vi "Main.vi"(11 "Module Admin":refnum<class "Delacor_lib_QMH_Cloneable Module Admin.lvclass">) -> ()   [LabVIEW 2020, in "Monochromator.lvlib"]
doc: "This template is based off of the Queued Message Handler design pattern and the Queued Message Handler project template that ships with LabVIEW.\n\nThe main difference is that the queue is private to this module and communication between modules is performed via Broadcast and Request events.\n\nRequest events are wrapped in public API methods and are handled in the Event Handling Loop (EHL) of this VI. Any module can register for Broadcast events sent by this module. The EHL generates messages based on user interface actions.\n\nThe Message Handling Loop (MHL) processes messages generated by the EHL, or by other messages. The messages are string values, so new messages can be added easily to the Message Cases case structure in the MHL. Each message cluster can also provide an optional value for Message Data, which is a variant that can be converted to whatever message-specific data is required.\n_____\nBased on DQMH Project Template 6.1.0.94.\n____\nPantherLAB Templates 1.0.0.1\nCopyright (c) 2022, PantherLAB\n____\nPantherLAB Templates 1.0.0.5\nCopyright (c) 2022, PantherLAB"
uses:
  Monochromator.lvlib
  <vilib>/Delacor/Delacor QMH/Libraries/Cloneable Module Admin_class/Delacor_lib_QMH_Cloneable Module Admin.lvclass
  C:/Program Files (x86)/National Instruments/LabVIEW 2020/vi.lib/Delacor/Delacor QMH/Libraries/Module Admin_class/Delacor_lib_QMH_Module Admin.lvclass
  Module Data--cluster.ctl
  <vilib>/Delacor/Delacor QMH/Libraries/Cloneable Module Admin_class/Delacor_lib_QMH_Cloneable Module Admin.lvclass/Delacor_lib_QMH_Cloneable Module Admin.ctl
  Helper Loop Status--enum.ctl
  <vilib>/Delacor/Delacor QMH/Libraries/Message Queue_class/Delacor_lib_QMH_Message Queue.lvclass/Delacor_lib_QMH_Message Queue.ctl
  Stop Argument--cluster.ctl
  <vilib>/Delacor/Delacor QMH/Libraries/Module Admin_class/Delacor_lib_QMH_Module Admin.lvclass/Delacor_lib_QMH_Module Admin.ctl
  Draw Panel into Subpanel Argument--cluster.ctl
  Remove Panel from Subpanel Argument--cluster.ctl
  Connect Argument--cluster.ctl
  Connect (Reply Payload)--cluster.ctl
  Move Argument--cluster.ctl
  Read continuously Argument--cluster.ctl
  Stop continous reading Argument--cluster.ctl
  Stop movement Argument--cluster.ctl
  Ask position Argument--cluster.ctl
  Ask position (Reply Payload)--cluster.ctl
  Position reached Argument--cluster.ctl
  Position reached (Reply Payload)--cluster.ctl
  Set speed Argument--cluster.ctl
  Get speed Argument--cluster.ctl
  Get speed (Reply Payload)--cluster.ctl
  Disconnect Argument--cluster.ctl
  Move (GOTO) Argument--cluster.ctl
  Move (GOTO) (Reply Payload)--cluster.ctl
  <vilib>/Utility/miscctls.llb/LVPointTypeDef.ctl
  Support/HL Data.ctl
  <vilib>/Instr/_visa.llb/VISA Flush IO Buffer Mask.ctl
  <vilib>/Delacor/Delacor QMH/Libraries/Cloneable Module Admin_class/Delacor_lib_QMH_Get Module ID.vi
  <vilib>/Delacor/Delacor QMH/Libraries/Message Queue_class/Delacor_lib_QMH_Enqueue Message (Single).vi
  <vilib>/Delacor/Delacor QMH/Libraries/Module Admin_class/Delacor_lib_QMH_Get External Launch.vi
  <vilib>/Utility/error.llb/Error Cluster From Error Code.vi
  <vilib>/ErrorRing/Error Ring.xnode
  <vilib>/Delacor/Delacor QMH/Libraries/Message Queue_class/Delacor_lib_QMH_Message Queue.lvclass
  Local Events/Local Events.lvlib
panel:
  out "error out":errorcluster
  out "Status":string
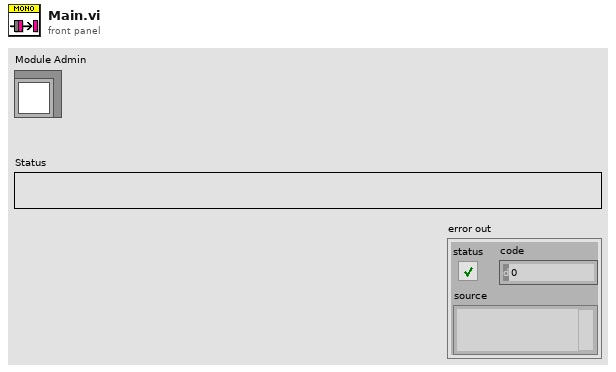
[diagram p1: front panel]
types:
  T1 = typedef "Monochromator.lvlib/Request Events--cluster.ctl" = cluster{"Stop Module":refnum<user-event>, "Show Panel":refnum<user-event>, "Hide Panel":refnum<user-event>, "Show Diagram":refnum<user-event>, "Get Module Execution Status":refnum<user-event>, "Draw Panel into Subpanel":refnum<user-event>, "Remove Panel from Subpanel":refnum<user-event>, "Connect":refnum<user-event>, "Move":refnum<user-event>, "Read continuously":refnum<user-event>, "Stop continous reading":refnum<user-event>, "Stop movement":refnum<user-event>, "Ask position":refnum<user-event>, "Position reached":refnum<user-event>, "Set speed":refnum<user-event>, "Get speed":refnum<user-event>, "Disconnect":refnum<user-event>, "Move (GOTO)":refnum<user-event>}
  T2 = typedef "Monochromator.lvlib/Local Events.lvlib/Local Events--cluster.ctl" = cluster{"Wake up Helper Loop":refnum<user-event>, "Put Helper Loop to Sleep":refnum<user-event>}
  T3 = typedef "Monochromator.lvlib/Module Data--cluster.ctl" = cluster{"Status":string, "SubPanel":refnum<vi>, "Panel Status":bool, "VISA resource name":refnum<visa-resource-name>, "Simulate?":bool, "Current position":dbl, "Current speed":dbl, "Connected?":bool, "Desired position":dbl}
  T4 = enum32{"invalid lock state", "Not Locked", "Locked (No Password)", "Password-protected"}
  T5 = typedef "Monochromator.lvlib/Stop Argument--cluster.ctl" = cluster{"Module ID":i32, "Origin":string, "Exit via Stop Module Req?":bool, "Wait for Module to stop?":bool}
  T6 = typedef "Monochromator.lvlib/Draw Panel into Subpanel Argument--cluster.ctl" = cluster{"Module ID":i32, "Sub Panel":refnum<vi>}
  T7 = typedef "Monochromator.lvlib/Remove Panel from Subpanel Argument--cluster.ctl" = cluster{"Module ID":i32, "Boolean":bool}
  T8 = typedef "Monochromator.lvlib/Connect Argument--cluster.ctl" = cluster{"Module ID":i32, "VISA resource name":refnum<visa-resource-name>, "Port config":cluster{"baud rate":u32, "data bits":u16, "parity":enum16{"None", "Odd", "Even", "Mark", "Space"}, "stop bits":u16}, "Wait Notifier":refnum<notifier>, "wait for reply":bool, "Simulate?":bool}
  T9 = typedef "Monochromator.lvlib/Move Argument--cluster.ctl" = cluster{"Module ID":i32, "Wavelength":dbl}
  T10 = typedef "Monochromator.lvlib/Read continuously Argument--cluster.ctl" = cluster{"Module ID":i32, "Timeout":i32}
  T11 = typedef "Monochromator.lvlib/Stop continous reading Argument--cluster.ctl" = cluster{"Module ID":i32, "Boolean":bool}
  T12 = typedef "Monochromator.lvlib/Stop movement Argument--cluster.ctl" = cluster{"Module ID":i32, "Boolean":bool}
  T13 = typedef "Monochromator.lvlib/Ask position Argument--cluster.ctl" = cluster{"Module ID":i32, "Wait Notifier":refnum<notifier>, "wait for reply":bool}
  T14 = typedef "Monochromator.lvlib/Position reached Argument--cluster.ctl" = cluster{"Module ID":i32, "Wait Notifier":refnum<notifier>, "wait for reply":bool}
  T15 = typedef "Monochromator.lvlib/Set speed Argument--cluster.ctl" = cluster{"Module ID":i32, "nm/min":dbl}
  T16 = typedef "Monochromator.lvlib/Get speed Argument--cluster.ctl" = cluster{"Module ID":i32, "Wait Notifier":refnum<notifier>, "wait for reply":bool}
  T17 = typedef "Monochromator.lvlib/Disconnect Argument--cluster.ctl" = cluster{"Module ID":i32, "Boolean":bool}
  T18 = typedef "Monochromator.lvlib/Move (GOTO) Argument--cluster.ctl" = cluster{"Module ID":i32, "Position":dbl, "Echo?":bool, "Wait Notifier":refnum<notifier>, "wait for reply":bool}
  T19 = typedef "LVPointTypeDef.ctl" = cluster{"Horizontal":i16, "Vertical":i16}
  T20 = enum32{"Invalid", "Standard", "Closed", "Hidden", "Minimized", "Maximized"}
  T21 = typedef "Monochromator.lvlib/Connect (Reply Payload)--cluster.ctl" = cluster{"Connected?":bool, "error":errorcluster}
  T22 = typedef "Monochromator.lvlib/Move (GOTO) (Reply Payload)--cluster.ctl" = cluster{"error":errorcluster}
  T23 = typedef "Monochromator.lvlib/HL Data.ctl" = cluster{"Helper Loop Timeout":i32, "VISA resource name":refnum<visa-resource-name>, "Module ID":i32}
  T24 = typedef "Monochromator.lvlib/Ask position (Reply Payload)--cluster.ctl" = cluster{"Current position":dbl, "error":errorcluster}
  T25 = typedef "Monochromator.lvlib/Position reached (Reply Payload)--cluster.ctl" = cluster{"Done?":bool, "error":errorcluster}
  T26 = typedef "Monochromator.lvlib/Get speed (Reply Payload)--cluster.ctl" = cluster{"nm/min":dbl, "error":errorcluster}
  T27 = typedef "Monochromator.lvlib/Helper Loop Status--enum.ctl" = enum16{"Awake", "Asleep"}
  T28 = cluster{"baud rate":u32, "data bits":u16, "parity":enum16{"None", "Odd", "Even", "Mark", "Space"}, "stop bits":u16}
  T29 = typedef "VISA Flush IO Buffer Mask.ctl" = u16
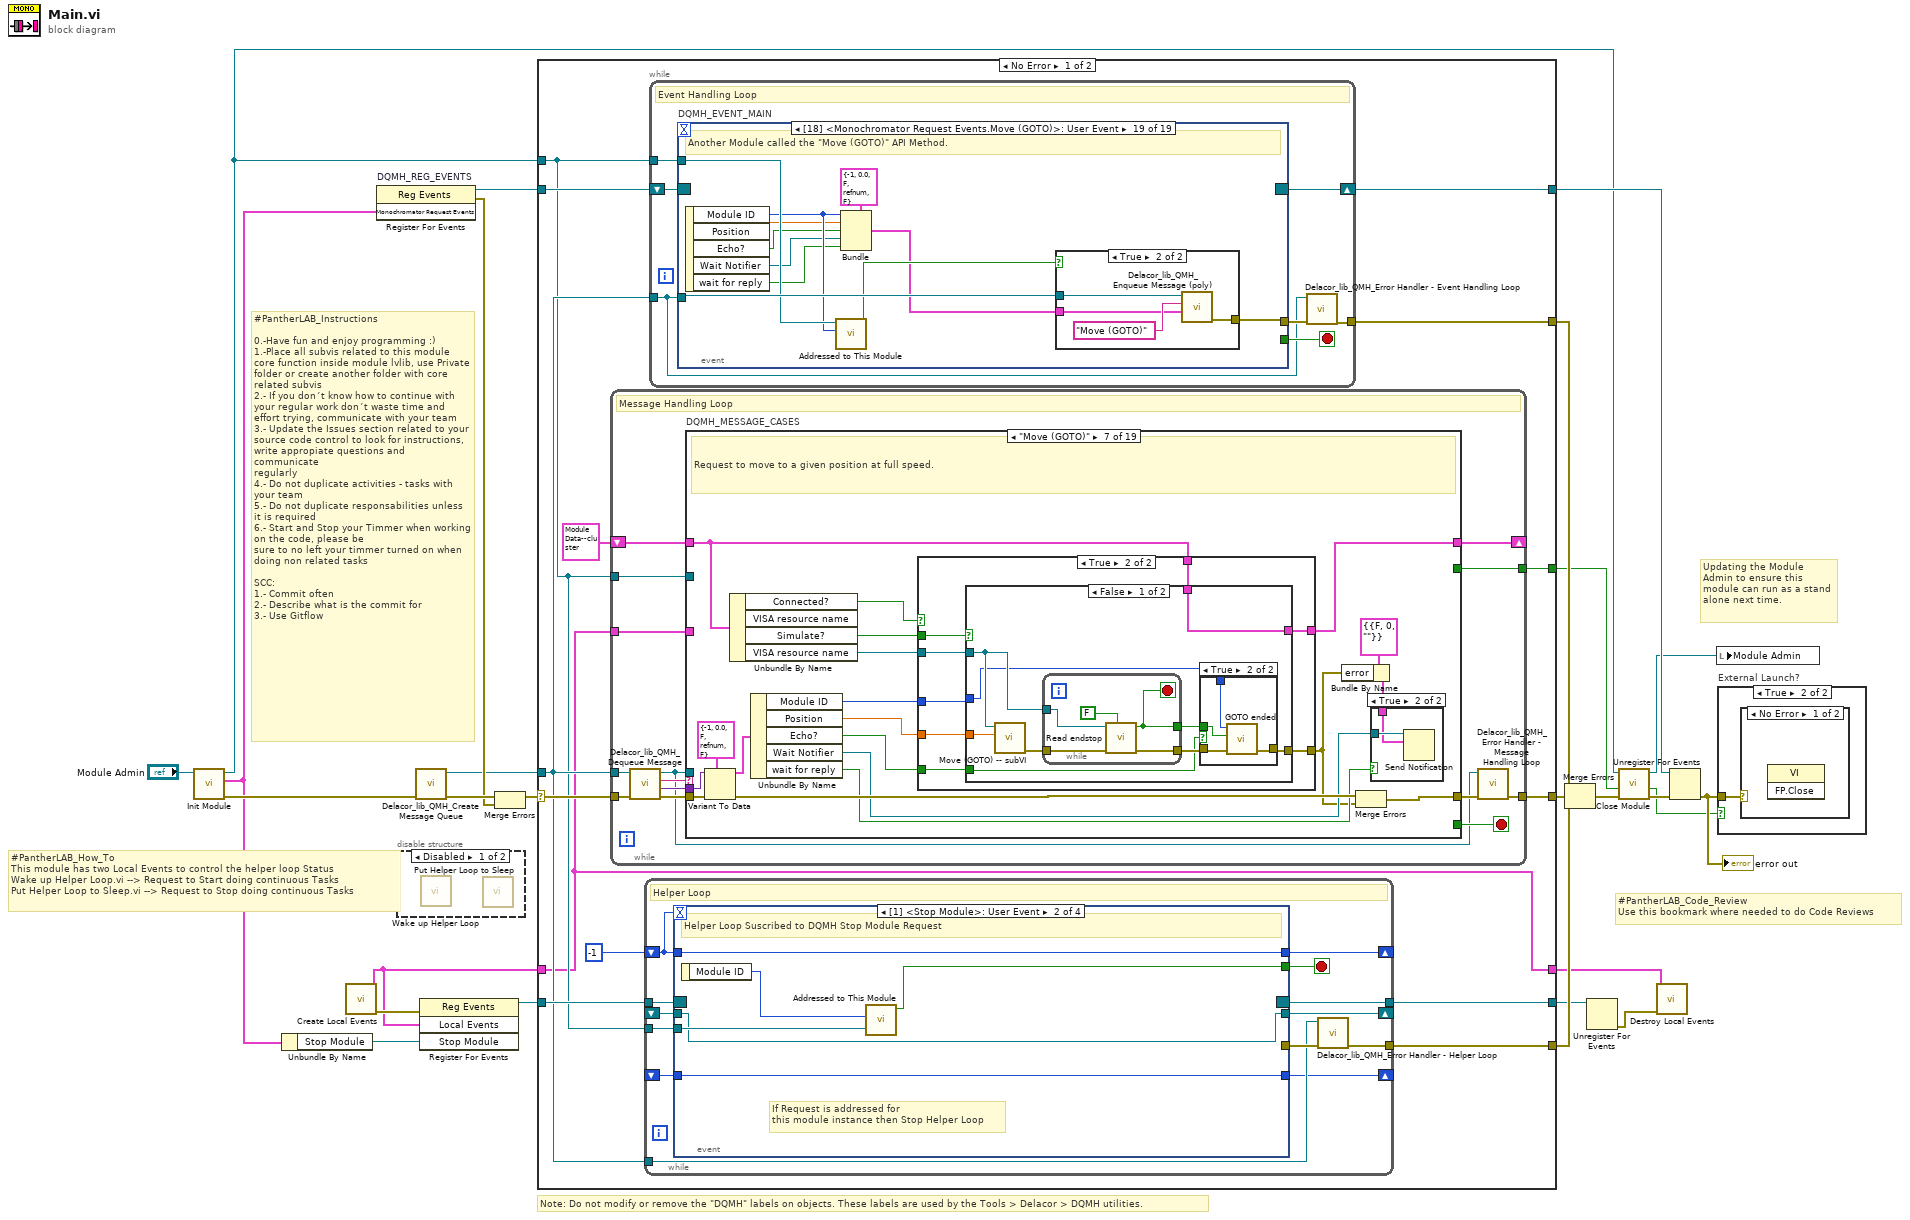
[diagram p0: block diagram]
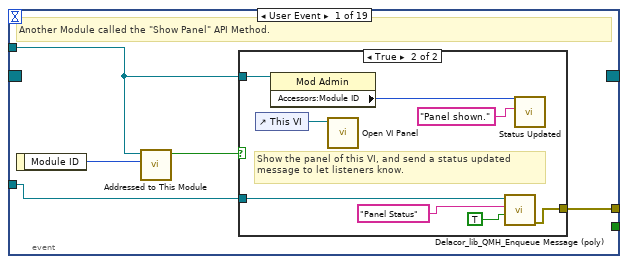
[diagram p2: hidden frame]
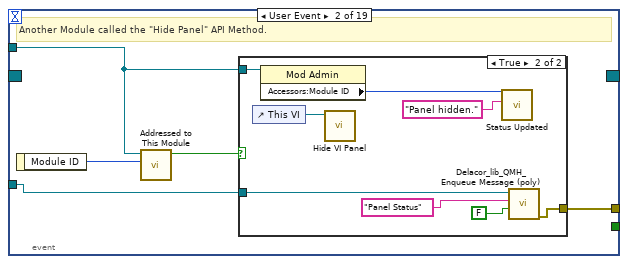
[diagram p4: hidden frame]
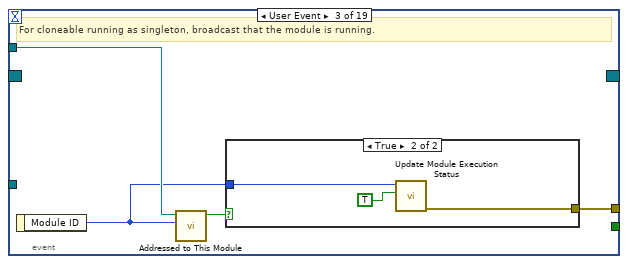
[diagram p6: hidden frame]
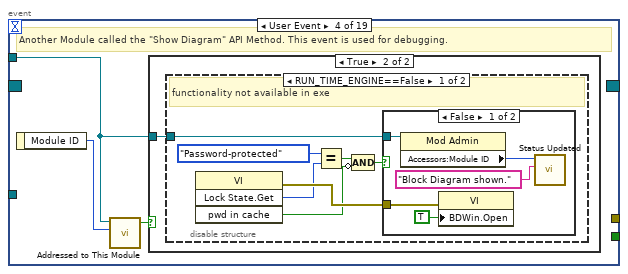
[diagram p8: hidden frame]
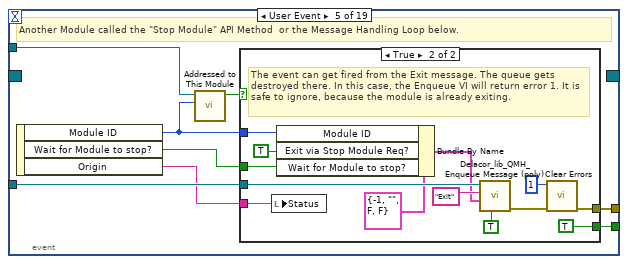
[diagram p12: hidden frame]
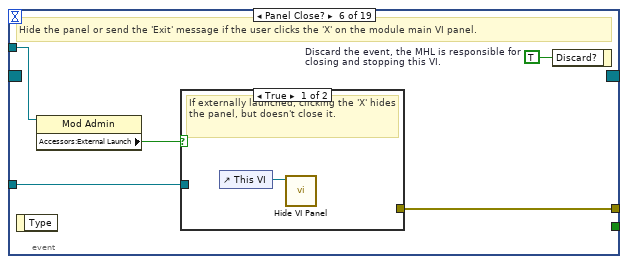
[diagram p14: hidden frame]
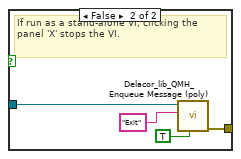
[diagram p15: hidden frame]
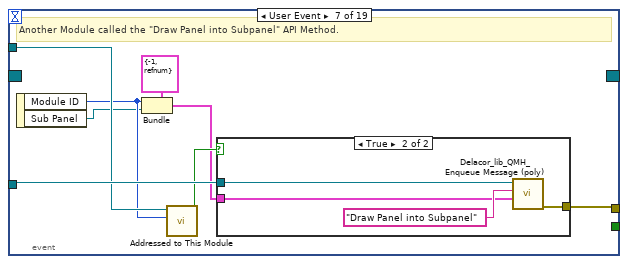
[diagram p16: hidden frame]
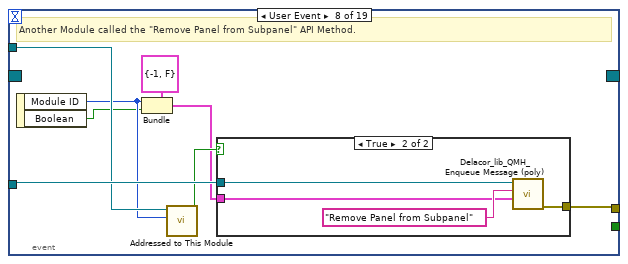
[diagram p18: hidden frame]
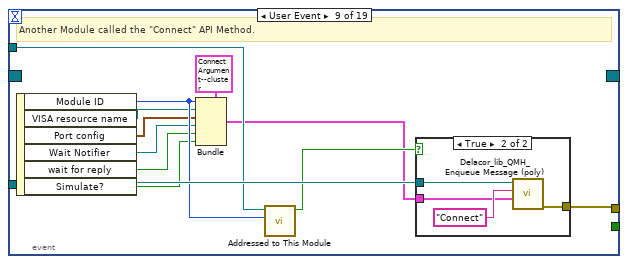
[diagram p20: hidden frame]
diagram:
  # "#PantherLAB_How_To\nThis module has two Local Events to control the helper loop Status\nWake up Helper Loop.vi --> Request to Start doing continuous Tasks\nPut Helper Loop to Sleep.vi --> Request to Stop doing continuous Tasks"
  # "#PantherLAB_Code_Review\nUse this bookmark where needed to do Code Reviews"
  # "#PantherLAB_Instructions\n\n0.-Have fun and enjoy programming :)\n1.-Place all subvis related to this module core function inside module lvlib, use Private folder or create another folder with core related subvis \n2.- If you don´t know how to continue with your regular work don´t waste time and effort trying, communicate with your team\n3.- Update the Issues section related to your source code control to look for instructions, write appropiate questions and communicate\nregularly\n4.- Do not duplicate activities - tasks with your team\n5.- Do not duplicate responsabilities unless it is required\n6.- Start and Stop your Timmer when working on the code, please be\nsure to no left your timmer turned on when doing non related tasks\n\nSCC:\n1.- Commit often\n2.- Describe what is the commit for\n3.- Use Gitflow"
  # "Note: Do not modify or remove the \"DQMH\" labels on objects. These labels are used by the Tools > Delacor > DQMH utilities."
  # "Updating the Module Admin to ensure this module can run as a stand alone next time."
  n1 = call "Init Module.vi"("Cloneable Module Admin in"="Module Admin") -> ("error out"=w23:errorcluster, "Monochromator Request Events"=w4:T1, "Cloneable Module Admin out"=w10:refnum<class "Delacor_lib_QMH_Cloneable Module Admin.lvclass">)  [unwired: 8 in]
  n2 = Unbundle By Name(w4) -> ("Stop Module"=w3:refnum<user-event>)
  n3 = call "Create Local Events.vi"() -> ("error out"=w16:errorcluster, "Local Events"=w2:T2)  [unwired: 10 in]
  n4 = register-events "DQMH_REG_EVENTS"(w4) -> (reference out=w13:refnum<event-registration>, error out=w18:errorcluster)  [unwired: 2 in]
  n5 = disable-structure shown="Disabled" {
    frame Disabled {
      n6 = call "Wake up Helper Loop.vi"() -> ()  [unwired: 11 in, 1 out]
      n7 = call "Put Helper Loop to Sleep.vi"() -> ()  [unwired: 11 in, 1 out]
    }
    frame Enabled {
    }
  }
  n8 = call <vilib>:"Delacor_lib_QMH_Create Message Queue.vi"("error in"=w23) -> ("error out"=w20:errorcluster, "Message Queue"=w12:refnum<class "Delacor_lib_QMH_Message Queue.lvclass">)  [unwired: 9 in]
  n9 = register-events(error in=w16, w2, w3) -> (reference out=w5:refnum<event-registration>)  [unwired: 1 in, 1 out]
  n10 = Merge Errors(w20, w18) -> (w19:errorcluster)
  n11 = case shown="No Error" w19 {
    selector: w19 -> [w38 w907]
    tunnel: [w40 w906] -> w24
    tunnel: [w36 w905] -> w14
    tunnel: w13 -> [w34 w905]
    tunnel: w12 -> [w29 w898]
    tunnel: [w39 _] -> w25
    tunnel: w10 -> [w28 w901]
    tunnel: [w33 _] -> w8
    tunnel: [w32 w897] -> w6
    tunnel: w5 -> [w31 w897]
    tunnel: [w37 _] -> w17
    tunnel: w2 -> [w27 w896]
    tunnel: [w27 w896] -> w1
    frame No Error {
      n12 = while {
        tunnel: w29 -> [w298]
        shift-right: [w302] -> _
        shift-left: T3 {"Status"="", "SubPanel"=refnum, "Panel Status"=FALSE, "VISA resource name"="", "Simulate?"=FALSE, "Current position"=0.0, "Current speed"=0.0, "Connected?"=FALSE, "Desired position"=0.0} ("Data Cluster") -> [w303]
        tunnel: w38 -> [w306]
        tunnel: [w304] -> w40
        tunnel: w28 -> [w296]
        tunnel: [w295] -> w33
        tunnel: w27 -> [w294]
        stop <- w301 stop-if-true
        # "Message Handling Loop"
        n13 = call-dynamic "Delacor_lib_QMH_Dequeue Message.vi"("error in"=w306, "Message Queue in"=w298) -> ("error out"=w305:errorcluster, "Message Data"=w299:variant, "Message"=w300:string, "Message Queue out"=w297:refnum<class "Delacor_lib_QMH_Message Queue.lvclass">)  [unwired: 6 in]
        n14 = case "DQMH_MESSAGE_CASES" shown="\"Move (GOTO)\"" w300 {
          selector: w300 -> [_ _ _ _ _ _ _ _ _ _ _ _ _ _ _ w772 _ _ _]
          tunnel: w297 -> [_ _ _ _ _ _ _ _ _ _ _ _ _ _ _ _ w786 w819 _]
          tunnel: w305 -> [w326 w335 w347 w366 w397 w423 w469 w522 w555 w569 w609 w654 w685 w727 w756 w774 w795 w824 w837]
          tunnel: [w324 w334 w345 w365 w388 w417 w460 w516 w550 w564 w600 w645 w679 w718 w750 w775 w791 w822 w837] -> w307
          tunnel: w303 -> [w317 w333 w338 w360 w385 w412 w457 w513 w548 w563 w593 w644 w676 w716 w752 w773 w790 w810 w836]
          tunnel: [w316 w330 w337 w360 w384 w411 w456 w513 w548 w563 w592 w644 w675 w716 w752 w773 w790 w810 w836] -> w302
          tunnel: [_ _ _ _ _ _ _ _ _ _ _ _ _ _ _ _ _ w818 _] -> w301
          tunnel: w299 -> [_ w332 w343 w364 w395 w422 w467 w521 w554 w568 w607 w652 w684 w725 w755 _ w789 w816 _]
          tunnel: w296 -> [w311 _ w336 w359 _ _ _ _ _ _ _ _ _ _ _ w770 w788 w812 _]
          tunnel: [_ _ _ _ _ _ _ _ _ _ _ _ _ _ _ _ _ w814 _] -> w295
          tunnel: w294 -> [_ _ _ _ _ _ _ w518 w549 _ _ _ _ _ _ _ _ _ _]
          frame "Initialize" {
            w308 = "Initial Message" ("Initial Message")
            # "#CodeNeeded - Initialize the appearance of the front panel."
            # "#CodeNeeded - Initialize your state data here."
            # "Initialize - Any operation that needs to be done before the module can receive messages. Synchronize Caller Events.vi will inform Start Module.vi that the module has launched and is ready to receive messages. Module Did Init.vi will broadcast that the module initialized."
            n15 = call "Synchronize Caller Events.vi"("error in (no error)"=w326, "Module Admin"=w311) -> ("error out"=w325:errorcluster, "Module Admin out"=w310:refnum<class "Delacor_lib_QMH_Cloneable Module Admin.lvclass">)  [unwired: 8 in]
            n16 = property class="Mod Admin"(reference=w310) -> ("Accessors:Module ID"=w313:i32, "Accessors:External Launch"=w312:bool)  [unwired: 1 in, 2 out]
            n17 = call "Module Name--constant.vi"("Module ID"=w313) -> ("Module Name"=w321:string)  [unwired: 10 in]
            n18 = property class="VI"("Front Panel.Title"=w321) -> (reference out=w323:refnum<vi>, error out=w328:errorcluster)  [unwired: 2 in]
            n19 = Select(t=T20."Hidden" ("State"), s=w312, f=T20."Standard" ("State")) -> (s? t:f=w318:T20)
            n20 = invoke class="VI" method="FP.Open"(reference=w323, error in=w328, "State"=w318) -> (reference out=w322:refnum<vi>, error out=w327:errorcluster)  [unwired: 2 in, 3 out]
            n21 = call "Module Name--constant.vi"("Module ID"=w313) -> ("Module Name"=w314:string)  [unwired: 10 in]
            n22 = Bundle By Name(cluster=w317, "Status"=w308) -> (w316:T3)
            n23 = invoke class="VI" method="FP.Center"(reference=w322, error in=w327) -> ()  [unwired: 1 in, 3 out]
            n24 = property on="Pane" class="Pane"("Origin"=T19 {"Horizontal"=0, "Vertical"=0}) -> ()  [unwired: 2 in, 2 out]
            n25 = call "Module Did Init.vi"("error in (no error)"=w325, "Initialized?"=TRUE, "Origin"=w314, "Module ID"=w313) -> ("error out"=w324:errorcluster)  [unwired: 7 in]
            "Status" <- w308
          }
          frame "Panel Status" {
            n26 = Variant To Data(error in=w335, type=TRUE, Variant=w332) -> (data=w329:bool, error out=w334:errorcluster)
            n27 = Bundle By Name(cluster=w333, "Panel Status"=w329) -> (w330:T3)
          }
          frame "Draw Panel into Subpanel" {
            # "Draw instance panel into panel provided"
            n28 = Variant To Data(error in=w347, type=T6 {"Module ID"=-1, "Sub Panel"=refnum} ("Draw Panel into Subpanel Argument"), Variant=w343) -> (data=w341:T6, error out=w346:errorcluster)
            n29 = Unbundle By Name(w341) -> ("Module ID"=w339:i32, "Sub Panel"=w340:refnum<vi>)
            n30 = case shown="Default" w339 {
              tunnel: w340 -> [_ w357]
              tunnel: [w352 w358] -> w344
              tunnel: w338 -> [w350 w355]
              tunnel: [w350 w354] -> w337
              tunnel: w336 -> [w349 _]
              frame Default {
                n31 = property class="Mod Admin"(reference=w349) -> ("Accessors:Module ID"=w348:i32)  [unwired: 1 in, 2 out]
                n32 = call "Status Updated.vi"("Status"="Please send \"Draw Panel into Subpanel\" Request to this Module ID Instance", "Module ID"=w348) -> ("error out"=w352:errorcluster)  [unwired: 9 in]
              }
              frame 0.. {
                n33 = control-ref of="This VI"() -> (w356:refnum<vi>)
                n34 = call "Draw Panel into Subpanel Procedure.vi"("SubPanel in"=w357, "This VI"=w356) -> ("error out"=w358:errorcluster, "SubPanel out"=w353:refnum<vi>)  [unwired: 8 in]
                n35 = Bundle By Name(cluster=w355, "SubPanel"=w353) -> (w354:T3)
              }
            }
            n36 = Merge Errors(w346, w344) -> (w345:errorcluster)
          }
          frame "Remove Panel from Subpanel" {
            # "Remove panel from subpanel"
            n37 = Variant To Data(error in=w366, type=T7 {"Module ID"=-1, "Boolean"=FALSE} ("Remove Panel from Subpanel Argument"), Variant=w364) -> (data=w362:T7, error out=w365:errorcluster)
            n38 = Unbundle By Name(w362) -> ("Module ID"=w361:i32)
            n39 = case shown="-1" w361 {
              tunnel: w360 -> [w370 _]
              tunnel: w359 -> [_ w374]
              frame Default {
                n40 = Unbundle By Name(w370) -> ("Panel Status"=w368:bool, "SubPanel"=w369:refnum<vi>)
                n41 = control-ref of="This VI"() -> (w367:refnum<vi>)
                n42 = case shown="True" w368 {
                  tunnel: w367 -> [w371 w372]
                  frame False {
                    n43 = call "Hide VI Panel.vi"("VI"=w371) -> ()  [unwired: 10 in, 1 out]
                  }
                  frame True {
                    n44 = call "Open VI Panel.vi"("VI"=w372) -> ()  [unwired: 10 in, 1 out]
                  }
                }
                n45 = invoke class="SubPnl" method="Remove VI"(reference=w369) -> ()  [unwired: 2 in, 3 out]
              }
              frame -1 {
                n46 = property class="Mod Admin"(reference=w374) -> ("Accessors:Module ID"=w373:i32)  [unwired: 1 in, 2 out]
                n47 = call "Status Updated.vi"("Status"="Please send \"Remove panel from subpanel\" Request to this Module ID Instance", "Module ID"=w373) -> ()  [unwired: 9 in, 1 out]
              }
            }
          }
          frame "Connect" {
            w376 = 0.0 ("Current position")
            # "Request to connect to a SP-2500i"
            n48 = Variant To Data(error in=w397, type=T8 {"Module ID"=-1, "VISA resource name"="", "Port config"={"baud rate"=9600, "data bits"=8, "parity"=enum."None", "stop bits"=10}, "Wait Notifier"=refnum, "wait for reply"=FALSE, "Simulate?"=FALSE} ("Connect Argument"), Variant=w395) -> (data=w393:T8, error out=w396:errorcluster)
            n49 = Unbundle By Name(w393) -> ("Simulate?"=w377:bool, "Module ID"=w379:i32, "VISA resource name"=w387:refnum<visa-resource-name>, "Port config"=w386:T28, "Wait Notifier"=w392:refnum<notifier>, "wait for reply"=w391:bool)
            n50 = call "Initialize.vi"("Simulate?"=w377, "Port config"=w386, "VISA Refnum in"=w387) -> ("error out"=w381:errorcluster, "Connected?"=w382:bool, "VISA Refnum out"=w383:refnum<visa-resource-name>)  [unwired: 6 in]
            n51 = case shown="False" w382 {
              selector: w382 -> [w403 w408]
              tunnel: w381 -> [w402 w407]
              tunnel: [w400 w406] -> w380
              tunnel: [w403 w408] -> w378
              tunnel: w379 -> [w399 w404]
              frame False {
                n52 = call <vilib>:"Clear Errors.vi"("error in (no error)"=w402) -> ("error out"=w401:errorcluster)  [unwired: 5 in, 1 out]
                n53 = call "Status Updated.vi"("error in (no error)"=w401, "Status"="Connection not successful.", "Module ID"=w399) -> ("error out"=w400:errorcluster)  [unwired: 8 in]
              }
              frame True {
                n54 = call "Status Updated.vi"("error in (no error)"=w407, "Status"="Connection successful.", "Module ID"=w404) -> ("error out"=w406:errorcluster)  [unwired: 8 in]
              }
            }
            n55 = Bundle By Name(cluster=T21 {"Connected?"=FALSE, "error"={"status"=FALSE, "code"=0, "source"=""}} ("Connect (Reply Payload)"), "Connected?"=w378, "error"=w380) -> (w390:T21)
            n56 = Bundle By Name(cluster=w385, "Desired position"=w376, "Current position"=w376, "Simulate?"=w377, "VISA resource name"=w383, "Connected?"=w378) -> (w384:T3)
            n57 = Merge Errors(w396, w380) -> (w388:errorcluster)
            n58 = case shown="True" w391 {
              tunnel: w392 -> [_ w410]
              tunnel: w390 -> [_ w409]
              frame False {
              }
              frame True {
                n59 = Send Notification(notification=w409, notifier=w410) -> ()  [unwired: 1 in, 2 out]
              }
            }
          }
          frame "Move" {
            # "Move to a specific wavelenght."
            n60 = Variant To Data(error in=w423, type=T9 {"Module ID"=-1, "Wavelength"=0.0} ("Move Argument"), Variant=w422) -> (data=w420:T9, error out=w419:errorcluster)
            n61 = Unbundle By Name(w412) -> ("Connected?"=w413:bool, "VISA resource name"=w418:refnum<visa-resource-name>, "Simulate?"=w416:bool)
            n62 = Unbundle By Name(w420) -> ("Module ID"=w415:i32, "Wavelength"=w414:dbl)
            n63 = case shown="False" w413 {
              tunnel: w419 -> [w427 w436]
              tunnel: w418 -> [_ w435]
              tunnel: [w428 w434] -> w417
              tunnel: w416 -> [_ w433]
              tunnel: w415 -> [w425 w432]
              tunnel: w414 -> [_ w431]
              tunnel: w412 -> [w424 w430]
              tunnel: [w424 w429] -> w411
              frame False {
                n64 = call "Status Updated.vi"("error in (no error)"=w427, "Status"="Device not connected. Cannot send commands.", "Module ID"=w425) -> ("error out"=w428:errorcluster)  [unwired: 8 in]
              }
              frame True {
                n65 = case shown="False" w433 {
                  tunnel: w436 -> [w441 w450]
                  tunnel: w435 -> [w440 _]
                  tunnel: w431 -> [w439 w442]
                  tunnel: [w438 w449] -> w434
                  tunnel: w432 -> [_ w448]
                  tunnel: w430 -> [w437 w444]
                  tunnel: [w437 w443] -> w429
                  frame False {
                    n66 = call "Move -- subVI.vi"("error in (no error)"=w441, "Wavelength"=w439, "VISA Refnum in"=w440) -> ("error out"=w438:errorcluster)  [unwired: 8 in]
                  }
                  frame True {
                    n67 = Format Into String(format string="%d nm", initial string="Simulating movement to ", w442) -> (resulting string=w445:string)  [unwired: 1 in, 1 out]
                    n68 = Bundle By Name(cluster=w444, "Desired position"=w442) -> (w443:T3)
                    n69 = call "Status Updated.vi"("error in (no error)"=w450, "Status"=w445, "Module ID"=w448) -> ("error out"=w449:errorcluster)  [unwired: 8 in]
                  }
                }
              }
            }
          }
          frame "Move (GOTO)" {
            # "Request to move to a given position at full speed."
            n70 = Variant To Data(error in=w469, type=T18 {"Module ID"=-1, "Position"=0.0, "Echo?"=FALSE, "Wait Notifier"=refnum, "wait for reply"=FALSE} ("Move (GOTO) Argument"), Variant=w467) -> (data=w465:T18, error out=w468:errorcluster)
            n71 = Unbundle By Name(w457) -> ("Connected?"=w455:bool, "Simulate?"=w454:bool, "VISA resource name"=w451:refnum<visa-resource-name>)  [unwired: 1 out]
            n72 = Unbundle By Name(w465) -> ("Module ID"=w459:i32, "Position"=w458:dbl, "Echo?"=w453:bool, "Wait Notifier"=w464:refnum<notifier>, "wait for reply"=w463:bool)
            n73 = case shown="True" w455 {
              tunnel: w451 -> [_ w481]
              tunnel: [w473 w480] -> w452
              tunnel: w454 -> [_ w479]
              tunnel: w459 -> [w471 w478]
              tunnel: w458 -> [_ w477]
              tunnel: w457 -> [w470 w476]
              tunnel: [w470 w475] -> w456
              tunnel: w453 -> [_ w474]
              frame False {
                n74 = call "Status Updated.vi"("Status"="Device not connected. Cannot send commands.", "Module ID"=w471) -> ("error out"=w473:errorcluster)  [unwired: 9 in]
              }
              frame True {
                n75 = case shown="False" w479 {
                  tunnel: w481 -> [w487 _]
                  tunnel: w477 -> [w490 w501]
                  tunnel: [w485 w508] -> w480
                  tunnel: w478 -> [w483 w507]
                  tunnel: w476 -> [w489 w503]
                  tunnel: [w489 w502] -> w475
                  tunnel: w474 -> [w482 _]
                  frame False {
                    n76 = call "Move (GOTO) -- subVI.vi"("Position"=w490, "VISA Refnum in"=w487) -> ("error out"=w488:errorcluster)  [unwired: 9 in]
                    n77 = while {
                      tunnel: w488 -> [w500]
                      tunnel: [w499] -> w486
                      tunnel: w487 -> [w498]
                      tunnel: [w496] -> w484
                      stop <- w496 stop-if-true
                      n78 = call "Read endstop.vi"("Simulate?"=FALSE, "error in (no error)"=w500, "VISA Refnum in"=w498) -> ("error out"=w499:errorcluster, "Done?"=w496:bool)  [unwired: 7 in]
                    }
                    n79 = case shown="True" w482 {
                      tunnel: w486 -> [w491 w495]
                      tunnel: [w491 w494] -> w485
                      tunnel: w484 -> [_ w493]
                      tunnel: w483 -> [_ w492]
                      frame False {
                      }
                      frame True {
                        n80 = call "GOTO ended.vi"("error in"=w495, "End?"=w493, "Module ID"=w492) -> ("error out"=w494:errorcluster)  [unwired: 8 in]
                      }
                    }
                  }
                  frame True {
                    n81 = Bundle By Name(cluster=w503, "Current position"=w501, "Desired position"=w501) -> (w502:T3)
                    n82 = Format Into String(format string="%d nm", initial string="Simulating movement to ", w501) -> (resulting string=w504:string)  [unwired: 1 in, 1 out]
                    n83 = call "Status Updated.vi"("Status"=w504, "Module ID"=w507) -> ("error out"=w508:errorcluster)  [unwired: 9 in]
                  }
                }
              }
            }
            n84 = Bundle By Name(cluster=T22 {"error"={"status"=FALSE, "code"=0, "source"=""}} ("Move (GOTO) (Reply Payload)"), "error"=w452) -> (w462:T22)
            n85 = Merge Errors(w468, w452) -> (w460:errorcluster)
            n86 = case shown="True" w463 {
              tunnel: w464 -> [_ w510]
              tunnel: w462 -> [_ w509]
              frame False {
              }
              frame True {
                n87 = Send Notification(notification=w509, notifier=w510) -> ()  [unwired: 1 in, 2 out]
              }
            }
          }
          frame "Read continuously" {
            # "Wake up the helper loop to read data from the port continuously."
            n88 = Variant To Data(error in=w522, type=T10 {"Module ID"=-1, "Timeout"=0} ("Read continuously Argument"), Variant=w521) -> (data=w519:T10, error out=w517:errorcluster)
            n89 = Unbundle By Name(w513) -> ("Connected?"=w511:bool, "Simulate?"=w512:bool)
            n90 = Unbundle By Name(w519) -> ("Timeout"=w515:i32, "Module ID"=w514:i32)
            n91 = case shown="False" w511 {
              tunnel: w518 -> [_ w533]
              tunnel: w517 -> [w525 w532]
              tunnel: [w526 w531] -> w516
              tunnel: w515 -> [_ w530]
              tunnel: w514 -> [w523 w529]
              tunnel: w513 -> [_ w528]
              tunnel: w512 -> [_ w527]
              frame False {
                n92 = call "Status Updated.vi"("error in (no error)"=w525, "Status"="Device not connected. Cannot send commands.", "Module ID"=w523) -> ("error out"=w526:errorcluster)  [unwired: 8 in]
              }
              frame True {
                n93 = case shown="False" w527 {
                  tunnel: w533 -> [w542 _]
                  tunnel: w532 -> [w541 w545]
                  tunnel: [w540 w546] -> w531
                  tunnel: w528 -> [w539 _]
                  tunnel: w530 -> [w538 _]
                  tunnel: w529 -> [w534 w544]
                  frame False {
                    n94 = Unbundle By Name(w539) -> ("VISA resource name"=w537:refnum<visa-resource-name>)
                    n95 = Bundle By Name(cluster=T23 {"Helper Loop Timeout"=0, "VISA resource name"="", "Module ID"=0} ("HL Data"), "VISA resource name"=w537, "Helper Loop Timeout"=w538, "Module ID"=w534) -> (w536:T23)
                    n96 = call "Wake up Helper Loop.vi"("error in"=w541, "HL Data"=w536, "Local Events"=w542) -> ("error out"=w540:errorcluster)  [unwired: 8 in]
                  }
                  frame True {
                    n97 = call "Status Updated.vi"("error in (no error)"=w545, "Status"="Cannot do continuous reading in simulated mode.", "Module ID"=w544) -> ("error out"=w546:errorcluster)  [unwired: 8 in]
                  }
                }
              }
            }
          }
          frame "Stop continous reading" {
            # "Request to stop continuous readings of the serial port."
            n98 = Variant To Data(error in=w555, type=T11 {"Module ID"=-1, "Boolean"=FALSE} ("Stop continous reading Argument"), Variant=w554) -> (data=w552:T11, error out=w551:errorcluster)
            n99 = Unbundle By Name(w548) -> ("Simulate?"=w547:bool)
            n100 = Unbundle By Name(w552) -> ()  [unwired: 1 out]
            n101 = case shown="False" w547 {
              tunnel: w551 -> [w558 w559]
              tunnel: [w557 w559] -> w550
              tunnel: w549 -> [w556 _]
              frame False {
                n102 = call "Put Helper Loop to Sleep.vi"("error in"=w558, "Local Events"=w556) -> ("error out"=w557:errorcluster)  [unwired: 9 in]
              }
              frame True {
              }
            }
          }
          frame "Stop movement" {
            # "Request to stop the movement of the monochromator."
            n103 = Variant To Data(error in=w569, type=T12 {"Module ID"=-1, "Boolean"=FALSE} ("Stop movement Argument"), Variant=w568) -> (data=w566:T12, error out=w565:errorcluster)
            n104 = Unbundle By Name(w563) -> ("Connected?"=w560:bool, "Simulate?"=w562:bool)
            n105 = Unbundle By Name(w566) -> ("Module ID"=w561:i32)
            n106 = case shown="True" w560 {
              tunnel: w565 -> [w573 w578]
              tunnel: [w572 w577] -> w564
              tunnel: w563 -> [_ w576]
              tunnel: w562 -> [_ w575]
              tunnel: w561 -> [w571 w574]
              frame False {
                n107 = call "Status Updated.vi"("error in (no error)"=w573, "Status"="Device not connected. Cannot send commands.", "Module ID"=w571) -> ("error out"=w572:errorcluster)  [unwired: 8 in]
              }
              frame True {
                n108 = case shown="False" w575 {
                  tunnel: w576 -> [w585 _]
                  tunnel: w578 -> [w584 w588]
                  tunnel: [w583 w589] -> w577
                  tunnel: w574 -> [_ w587]
                  frame False {
                    n109 = Unbundle By Name(w585) -> ("VISA resource name"=w582:refnum<visa-resource-name>)
                    n110 = Concatenate Strings("MONO-STOP" ("string"), "\r") -> (w581:string)
                    n111 = VISA Write(VISA resource name=w582, write buffer=w581, error in (no error)=w584) -> (error out=w583:errorcluster)  [unwired: 2 out]
                  }
                  frame True {
                    n112 = call "Status Updated.vi"("error in (no error)"=w588, "Status"="Simulating stop signal.", "Module ID"=w587) -> ("error out"=w589:errorcluster)  [unwired: 8 in]
                  }
                }
              }
            }
          }
          frame "Ask position" {
            # "Request to ask the current position of the monochromator."
            n113 = Unbundle By Name(w593) -> ("Connected?"=w595:bool, "Simulate?"=w597:bool, "VISA resource name"=w598:refnum<visa-resource-name>, "Desired position"=w590:dbl, "Current position"=w596:dbl)
            n114 = Variant To Data(error in=w609, type=T13 {"Module ID"=-1, "Wait Notifier"=refnum, "wait for reply"=FALSE} ("Ask position Argument"), Variant=w607) -> (data=w605:T13, error out=w608:errorcluster)
            n115 = Unbundle By Name(w605) -> ("Module ID"=w594:i32, "Wait Notifier"=w604:refnum<notifier>, "wait for reply"=w603:bool)
            n116 = case shown="True" w595 {
              tunnel: [w613 w619] -> w591
              tunnel: [w612 w618] -> w599
              tunnel: w598 -> [_ w617]
              tunnel: w597 -> [_ w616]
              tunnel: w596 -> [w613 w615]
              tunnel: w594 -> [w611 _]
              tunnel: w590 -> [_ w614]
              frame False {
                n117 = call "Status Updated.vi"("Status"="Device not connected. Cannot send commands.", "Module ID"=w611) -> ("error out"=w612:errorcluster)  [unwired: 9 in]
              }
              frame True {
                n118 = case shown="False" w616 {
                  selector: w616 -> [w620 _]
                  tunnel: [w623 w633] -> w619
                  tunnel: [w622 _] -> w618
                  tunnel: w617 -> [w621 _]
                  tunnel: w615 -> [_ w628]
                  tunnel: w614 -> [_ w629]
                  frame False {
                    n119 = call "Read position -- subVI.vi"("Simulate?"=w620, "VISA Refnum in"=w621) -> ("error out"=w622:errorcluster, "Current position"=w623:dbl)  [unwired: 8 in]
                  }
                  frame True {
                    n120 = Equal?(x=w629, y=w628) -> (x = y?=w632:bool)
                    n121 = Select(t=0.0, s=w632, f=10.0) -> (s? t:f=w625:dbl)
                    n122 = Greater Or Equal?(x=w629, y=w628) -> (x >= y?=w626:bool)
                    n123 = Select(t=w625, s=w626, f=-10.0) -> (s? t:f=w627:dbl)
                    n124 = Add(x=w627, y=w628) -> (x+y=w633:dbl)
                  }
                }
              }
            }
            n125 = Bundle By Name(cluster=T24 {"Current position"=0.0, "error"={"status"=FALSE, "code"=0, "source"=""}} ("Ask position (Reply Payload)"), "Current position"=w591, "error"=w599) -> (w602:T24)
            n126 = Bundle By Name(cluster=w593, "Current position"=w591) -> (w592:T3)
            n127 = Merge Errors(w608, w599) -> (w600:errorcluster)
            n128 = case shown="True" w603 {
              tunnel: w604 -> [_ w635]
              tunnel: w602 -> [_ w634]
              frame False {
              }
              frame True {
                n129 = Send Notification(notification=w634, notifier=w635) -> ()  [unwired: 1 in, 2 out]
              }
            }
          }
          frame "Position reached" {
            # "Request wheter the final position has been reached."
            n130 = Variant To Data(error in=w654, type=T14 {"Module ID"=-1, "Wait Notifier"=refnum, "wait for reply"=FALSE} ("Position reached Argument"), Variant=w652) -> (data=w650:T14, error out=w653:errorcluster)
            n131 = Unbundle By Name(w644) -> ("Current position"=w637:dbl, "Desired position"=w636:dbl, "Connected?"=w639:bool, "Simulate?"=w640:bool, "VISA resource name"=w643:refnum<visa-resource-name>)
            n132 = Unbundle By Name(w650) -> ("Module ID"=w638:i32, "Wait Notifier"=w649:refnum<notifier>, "wait for reply"=w648:bool)
            n133 = case shown="True" w639 {
              tunnel: w643 -> [_ w663]
              tunnel: [_ w662] -> w642
              tunnel: [w655 w661] -> w641
              tunnel: w640 -> [_ w660]
              tunnel: w638 -> [w656 _]
              tunnel: w637 -> [_ w659]
              tunnel: w636 -> [_ w658]
              frame False {
                n134 = call "Status Updated.vi"("Status"="Device not connected. Cannot send commands.", "Module ID"=w656) -> ("error out"=w655:errorcluster)  [unwired: 9 in]
              }
              frame True {
                n135 = case shown="False" w660 {
                  selector: w660 -> [w664 _]
                  tunnel: w663 -> [w667 _]
                  tunnel: [w666 w668] -> w662
                  tunnel: [w665 _] -> w661
                  tunnel: w659 -> [_ w670]
                  tunnel: w658 -> [_ w669]
                  frame False {
                    n136 = call "Read endstop.vi"("Simulate?"=w664, "VISA Refnum in"=w667) -> ("error out"=w665:errorcluster, "Done?"=w666:bool)  [unwired: 8 in]
                  }
                  frame True {
                    n137 = Greater Or Equal?(x=w670, y=w669) -> (x >= y?=w668:bool)
                  }
                }
              }
            }
            n138 = Merge Errors(w653, w641) -> (w645:errorcluster)
            n139 = Bundle By Name(cluster=T25 {"Done?"=FALSE, "error"={"status"=FALSE, "code"=0, "source"=""}} ("Position reached (Reply Payload)"), "Done?"=w642, "error"=w641) -> (w647:T25)
            n140 = case shown="True" w648 {
              tunnel: w649 -> [_ w672]
              tunnel: w647 -> [_ w671]
              frame False {
              }
              frame True {
                n141 = Send Notification(notification=w671, notifier=w672) -> ()  [unwired: 1 in, 2 out]
              }
            }
          }
          frame "Set speed" {
            # "Request to change speed in nm/min."
            n142 = Unbundle By Name(w676) -> ("VISA resource name"=w677:refnum<visa-resource-name>, "Simulate?"=w681:bool, "Connected?"=w673:bool)
            n143 = Variant To Data(error in=w685, type=T15 {"Module ID"=-1, "nm/min"=0.0} ("Set speed Argument"), Variant=w684) -> (data=w682:T15, error out=w680:errorcluster)
            n144 = Unbundle By Name(w682) -> ("Module ID"=w678:i32, "nm/min"=w674:dbl)
            n145 = case shown="True" w673 {
              tunnel: w681 -> [_ w695]
              tunnel: w680 -> [w688 w694]
              tunnel: [w689 w693] -> w679
              tunnel: w678 -> [w687 w692]
              tunnel: w677 -> [_ w691]
              tunnel: w674 -> [_ w690]
              frame False {
                n146 = call "Status Updated.vi"("error in (no error)"=w688, "Status"="Device not connected. Cannot send commands.", "Module ID"=w687) -> ("error out"=w689:errorcluster)  [unwired: 8 in]
              }
              frame True {
                n147 = case shown="False" w695 {
                  tunnel: w694 -> [w699 w711]
                  tunnel: [w698 w710] -> w693
                  tunnel: w692 -> [_ w709]
                  tunnel: w690 -> [w696 w706]
                  tunnel: w691 -> [w697 _]
                  frame False {
                    n148 = Format Into String(format string="%0.2f ", w696) -> (resulting string=w700:string)  [unwired: 2 in, 1 out]
                    n149 = Concatenate Strings(w700, "NM/MIN" ("string"), "\r") -> (w704:string)
                    n150 = VISA Write(VISA resource name=w697, write buffer=w704, error in (no error)=w699) -> (error out=w698:errorcluster)  [unwired: 2 out]
                  }
                  frame True {
                    n151 = Format Into String(format string="%d nm/min", initial string="Simulating speed of ", w706) -> (resulting string=w705:string)  [unwired: 1 in, 1 out]
                    n152 = call "Status Updated.vi"("error in (no error)"=w711, "Status"=w705, "Module ID"=w709) -> ("error out"=w710:errorcluster)  [unwired: 8 in]
                  }
                }
              }
            }
            n153 = Bundle By Name(cluster=w676, "Current speed"=w674) -> (w675:T3)
          }
          frame "Get speed" {
            # "Request to get the current speed in nm/min"
            n154 = Variant To Data(error in=w727, type=T16 {"Module ID"=-1, "Wait Notifier"=refnum, "wait for reply"=FALSE} ("Get speed Argument"), Variant=w725) -> (data=w723:T16, error out=w726:errorcluster)
            n155 = Unbundle By Name(w716) -> ("Simulate?"=w717:bool, "Connected?"=w713:bool)
            n156 = Unbundle By Name(w723) -> ("Module ID"=w712:i32, "Wait Notifier"=w722:refnum<notifier>, "wait for reply"=w721:bool)
            n157 = case shown="False" w713 {
              tunnel: w717 -> [_ w734]
              tunnel: w716 -> [_ w733]
              tunnel: [_ w732] -> w715
              tunnel: [w730 w731] -> w714
              tunnel: w712 -> [w729 _]
              frame False {
                n158 = call "Status Updated.vi"("Status"="Device not connected. Cannot send commands.", "Module ID"=w729) -> ("error out"=w730:errorcluster)  [unwired: 9 in]
              }
              frame True {
                n159 = case shown="False" w734 {
                  selector: w734 -> [w735 _]
                  tunnel: w733 -> [w739 w741]
                  tunnel: [w737 w740] -> w732
                  tunnel: [w736 _] -> w731
                  frame False {
                    n160 = Unbundle By Name(w739) -> ("VISA resource name"=w738:refnum<visa-resource-name>)
                    n161 = call "Read speed.vi"("Simulate?"=w735, "VISA Refnum in"=w738) -> ("error out"=w736:errorcluster, "number"=w737:dbl)  [unwired: 8 in]
                  }
                  frame True {
                    n162 = Unbundle By Name(w741) -> ("Current speed"=w740:dbl)
                  }
                }
              }
            }
            n163 = Merge Errors(w726, w714) -> (w718:errorcluster)
            n164 = Bundle By Name(cluster=T26 {"nm/min"=0.0, "error"={"status"=FALSE, "code"=0, "source"=""}} ("Get speed (Reply Payload)"), "nm/min"=w715, "error"=w714) -> (w720:T26)
            n165 = case shown="True" w721 {
              tunnel: w722 -> [_ w743]
              tunnel: w720 -> [_ w742]
              frame False {
              }
              frame True {
                n166 = Send Notification(notification=w742, notifier=w743) -> ()  [unwired: 1 in, 2 out]
              }
            }
          }
          frame "Disconnect" {
            # "Request to close connection with device."
            n167 = Unbundle By Name(w752) -> ("Simulate?"=w749:bool, "Connected?"=w748:bool, "VISA resource name"=w744:refnum<visa-resource-name>)
            n168 = Variant To Data(error in=w756, type=T17 {"Module ID"=-1, "Boolean"=FALSE} ("Disconnect Argument"), Variant=w755) -> (data=w753:T17, error out=w751:errorcluster)
            n169 = Unbundle By Name(w753) -> ("Module ID"=w745:i32)
            n170 = Not(x=w749) -> (.not. x?=w746:bool)
            n171 = And(x=w746, y=w748) -> (x .and. y?=w747:bool)
            n172 = case shown="True" w747 {
              tunnel: w751 -> [w757 w758]
              tunnel: [w757 w768] -> w750
              tunnel: w745 -> [_ w767]
              tunnel: w744 -> [_ w763]
              frame False {
              }
              frame True {
                w759 = T29 128 items=["Flush Receive Buffer"=16, "Write Transmit Buffer to Device"=32, "Flush Receive Buffer (No I/O)"=64, "Flush Transmit Buffer"=128] ("Mask")
                w760 = T29 64 items=["Flush Receive Buffer"=16, "Write Transmit Buffer to Device"=32, "Flush Receive Buffer (No I/O)"=64, "Flush Transmit Buffer"=128] ("Mask")
                n173 = Or(x=w760, y=w759) -> (x .or. y?=w761:T29)
                n174 = VISA Flush I/O Buffer(VISA resource name=w763, mask (16)=w761, error in (no error)=w758) -> (VISA resource name out=w762:refnum<visa-resource-name>, error out=w764:errorcluster)
                n175 = VISA Close(VISA resource name=w762, error in (no error)=w764) -> (error out=w766:errorcluster)
                n176 = call "Status Updated.vi"("error in (no error)"=w766, "Status"="Device disconnected.", "Module ID"=w767) -> ("error out"=w768:errorcluster)  [unwired: 8 in]
              }
            }
          }
          frame Default {
            # "'Default' case only runs if there is a message that isn't defined in any of the other cases.  Output a programming error."
            n177 = property class="Mod Admin"(reference=w770) -> ("Accessors:Module ID"=w769:i32)  [unwired: 1 in, 2 out]
            n178 = call "Module Name--constant.vi"("Module ID"=w769) -> ("Module Name"=w771:string)  [unwired: 10 in]
            n179 = xnode "Error Ring"("parameter 0"=w772, "parameter 1"=w771) -> ("error out"=w776:errorcluster)
            n180 = Merge Errors(w774, w776) -> (w775:errorcluster)
          }
          frame "Error" {
            # "#CodeRecommended - If you ever change the name of this \"Error\" message, you'll need to update the name in the Check Loop Error.vi as well."
            # "#CodeRecommended - If the module is running in standalone mode (External Launch = FALSE), this code will pop up an error dialog and call the 'Exit' message if an error occurs. Add more fine-grained error handling here."
            # "Error - Check the error message data and respond accordingly. This message is sent by the \"Error Handler\" VIs at the end of each loop in this application."
            n181 = property class="Mod Admin"(reference=w788) -> ("Accessors:External Launch"=w787:bool, "Accessors:Module ID"=w785:i32)  [unwired: 1 in, 2 out]
            n182 = Variant To Data(error in=w795, type=errorcluster {"status"=FALSE, "code"=0, "source"=""} ("error constant"), Variant=w789) -> (data=w796:errorcluster, error out=w793:errorcluster)
            n183 = call "Error Reported.vi"("Error"=w796, "Module ID"=w785) -> ()  [unwired: 9 in, 1 out]
            n184 = case shown="False" w787 {
              tunnel: [w801 _] -> w792
              tunnel: w786 -> [w799 _]
              tunnel: w796 -> [w800 _]
              frame False {
                # "If the module is running standalone, then pop up an error dialog and call the \"Exit\" message."
                n185 = call <vilib>:"Simple Error Handler.vi"("error in (no error)"=w800) -> ()  [unwired: 4 in, 5 out]
                n186 = call-poly <vilib>:"Delacor_lib_QMH_Enqueue Message (poly).vi"("Priority Message? (F)"=TRUE, "Message"="Exit", "Message Queue in"=w799) -> ("error out"=w801:errorcluster)  [unwired: 7 in, 1 out]
              }
              frame True {
                # "If the module was launched externally, calling the Error Reported broadcast VI is the only action performed by the \"Error\" message. The module's caller can then process the error appropriately."
              }
            }
            n187 = Merge Errors(w793, w792) -> (w791:errorcluster)
            n188 = local write "error out"(w791) -> ()
          }
          frame "Exit" {
            w818 = TRUE  # Stop the VI
            # "Exit - Exit the application."
            n189 = Variant To Data(error in=w824, type=T5 {"Module ID"=-1, "Origin"="", "Exit via Stop Module Req?"=FALSE, "Wait for Module to stop?"=FALSE} ("Stop Argument"), Variant=w816) -> (data=w813:T5, error out=w820:errorcluster)
            n190 = Unbundle By Name(w810) -> ("SubPanel"=w809:refnum<vi>, "VISA resource name"=w806:refnum<visa-resource-name>, "Simulate?"=w803:bool, "Connected?"=w805:bool)
            n191 = call <vilib>:"Clear Errors.vi"("error in (no error)"=w820, "specific error code to clear (0: all)"=91 ("91: not all Exit messages will have an argument")) -> ("error out"=w823:errorcluster)  [unwired: 4 in, 1 out]
            n192 = call-dynamic "Delacor_lib_QMH_Release Message Queue.vi"("error in"=w823, "Message Queue"=w819) -> ("error out"=w808:errorcluster)  [unwired: 9 in]
            n193 = Not(x=w803) -> (.not. x?=w802:bool)
            n194 = And(x=w802, y=w805) -> (x .and. y?=w804:bool)
            n195 = control-ref of="This VI"() -> (w811:refnum<vi>)
            n196 = case shown="True" w804 {
              tunnel: w808 -> [w825 w835]
              tunnel: [w825 w834] -> w807
              tunnel: w806 -> [_ w830]
              frame False {
              }
              frame True {
                w832 = T29 128 items=["Flush Receive Buffer"=16, "Write Transmit Buffer to Device"=32, "Flush Receive Buffer (No I/O)"=64, "Flush Transmit Buffer"=128] ("Mask")
                w833 = T29 16 items=["Flush Receive Buffer"=16, "Write Transmit Buffer to Device"=32, "Flush Receive Buffer (No I/O)"=64, "Flush Transmit Buffer"=128] ("Mask")
                n197 = Or(x=w833, y=w832) -> (x .or. y?=w831:T29)
                n198 = VISA Flush I/O Buffer(VISA resource name=w830, mask (16)=w831, error in (no error)=w835) -> (VISA resource name out=w829:refnum<visa-resource-name>, error out=w828:errorcluster)
                n199 = call "wait -- mono.vi"("error in (no error)"=w828, "milliseconds to wait"=u32 100) -> ("error out"=w827:errorcluster)  [unwired: 9 in]
                n200 = VISA Close(VISA resource name=w829, error in (no error)=w827) -> (error out=w834:errorcluster)
              }
            }
            n201 = call "Handle Exit.vi"("Stop Argument"=w813, "Module Admin in"=w812, "VI reference"=w811) -> ("error out"=w821:errorcluster, "Wait for Stop?"=w814:bool)  [unwired: 7 in]
            n202 = invoke class="SubPnl" method="Remove VI"(reference=w809) -> ()  [unwired: 2 in, 3 out]
            n203 = Merge Errors(w807, w821) -> (w822:errorcluster)
          }
          frame "---Exit and Error Handling---" {
            # "Separator - the following cases handle errors and exit messages."
          }
        }
        n204 = call-dynamic "Delacor_lib_QMH_Error Handler - Message Handling Loop.vi"("error in"=w307, "Message Queue in"=w297) -> ("dup error in"=w304:errorcluster)  [unwired: 8 in, 1 out]
      }
      n205 = while {
        tunnel: w29 -> [w844]
        tunnel: w31 -> [w848]
        shift-right: [w846] -> _
        shift-left: -1 ("Helper Loop Timeout") -> [w847]
        tunnel: [w845] -> w32
        tunnel: [w850] -> w37
        tunnel: w28 -> [w842]
        shift-right: [w841] -> _
        shift-left: _ -> [w840]
        shift-right: [w839] -> _
        shift-left: _ -> [w838]
        stop <- w843 stop-if-true
        # "Helper Loop"
        n206 = event shown="[1] <Stop Module>: User Event" {
          selector: w848 -> [_ _ _ _]
          dyn-events: [_ _ _ _] -> w845
          timeout: w847 -> [_ _ _ _]
          tunnel: w847 -> [w857 w881 _ _]
          tunnel: [w857 w881 w884 -1 ("Helper Loop Timeout")] -> w846
          tunnel: [_ w878 _ _] -> w843
          tunnel: w842 -> [w853 w880 w887 w894]
          tunnel: [w855 _ w888 w895] -> w849
          tunnel: [w851 w876 w883 w889] -> w841
          tunnel: w840 -> [w856 w876 _ w889]
          tunnel: [w852 w877 w882 w890] -> w839
          tunnel: w838 -> [w852 w877 _ w890]
          event Timeout {
            # "Continuous Tasks"
            n207 = event-data() -> ()  [unwired: 1 in, 1 out]
            n208 = call "Addressed to This Module.vi"("Module ID from Argument"=w852, "Module Admin"=w853) -> ("Addressed to this instance?"=w854:bool)  [unwired: 8 in, 1 out]
            n209 = case shown="True" w854 {
              tunnel: w856 -> [w858 w870]
              tunnel: [_ w865] -> w855
              tunnel: w853 -> [_ w864]
              tunnel: [w858 w859] -> w851
              frame False {
              }
              frame True {
                n210 = property class="Instr"(reference=w870) -> (reference out=w869:refnum<visa-resource-name>, error out=w868:errorcluster, "Bytes at Port"=w867:u32)  [unwired: 1 in]
                n211 = property class="Mod Admin"(reference=w864) -> ("Accessors:Module ID"=w863:i32)  [unwired: 1 in, 2 out]
                n212 = VISA Read(VISA resource name=w869, byte count=w867, error in (no error)=w868) -> (VISA resource name out=w859:refnum<visa-resource-name>, read buffer=w860:string, error out=w866:errorcluster)  [unwired: 1 out]
                n213 = Empty String/Path?(string/path=w860) -> (empty?=w862:bool)
                n214 = Not(x=w862) -> (.not. x?=w861:bool)
                n215 = case shown="True" w861 {
                  tunnel: w866 -> [w871 w875]
                  tunnel: [w871 w874] -> w865
                  tunnel: w863 -> [_ w873]
                  tunnel: w860 -> [_ w872]
                  frame False {
                  }
                  frame True {
                    # "String not empty. Broadcast."
                    n216 = call "Data read.vi"("error in"=w875, "Data read"=w872, "Module ID"=w873) -> ("error out"=w874:errorcluster)  [unwired: 8 in]
                  }
                }
              }
            }
          }
          event User Event {
            # "If Request is addressed for\nthis module instance then Stop Helper Loop"
            # "Helper Loop Suscribed to DQMH Stop Module Request"
            n217 = event-data() -> ("Module ID"=w879:i32)  [unwired: 1 in]
            n218 = call "Addressed to This Module.vi"("Module ID from Argument"=w879, "Module Admin"=w880) -> ("Addressed to this instance?"=w878:bool)  [unwired: 8 in, 1 out]
          }
          event User Event {
            # "Wake up Helper Loop, Start Continuous Tasks"
            n219 = event-data() -> ("Helper Loop Timeout"=w884:i32, "VISA resource name"=w883:refnum<visa-resource-name>, "Module ID"=w882:i32)  [unwired: 1 in]
            n220 = property class="Mod Admin"(reference=w887) -> ("Accessors:Module ID"=w885:i32)  [unwired: 1 in, 2 out]
            n221 = call "Helper Loop Status Updated.vi"("Helper Loop Status"=Helper_Loop_Status--enum."Awake", "Module ID"=w885) -> ("error out"=w888:errorcluster)  [unwired: 9 in]
          }
          event User Event {
            # "Put Helper Loop to Sleep"
            n222 = event-data() -> ()  [unwired: 1 in, 1 out]
            n223 = property class="Mod Admin"(reference=w894) -> ("Accessors:Module ID"=w891:i32)  [unwired: 1 in, 2 out]
            n224 = call "Helper Loop Status Updated.vi"("Helper Loop Status"=Helper_Loop_Status--enum."Asleep", "Module ID"=w891) -> ("error out"=w895:errorcluster)  [unwired: 9 in]
          }
        }
        n225 = call-dynamic "Delacor_lib_QMH_Error Handler - Helper Loop.vi"("error in"=w849, "Message Queue in"=w844) -> ("dup error in"=w850:errorcluster)  [unwired: 8 in, 1 out]
      }
      n226 = while {
        tunnel: w29 -> [w41]
        shift-right: [w44] -> w36
        shift-left: w34 -> [w45]
        tunnel: [w46] -> w39
        tunnel: w28 -> [w42]
        stop <- w43 stop-if-true
        # "Event Handling Loop"
        n227 = event "DQMH_EVENT_MAIN" shown="[18] <Monochromator Request Events.Move (GOTO)>: User Event" {
          selector: w45 -> [_ _ _ _ _ _ _ _ _ _ _ _ _ _ _ _ _ _ _]
          dyn-events: [_ _ _ _ _ _ _ _ _ _ _ _ _ _ _ _ _ _ _] -> w44
          timeout: _ -> [_ _ _ _ _ _ _ _ _ _ _ _ _ _ _ _ _ _ _]
          tunnel: [_ _ _ _ w100 _ _ _ _ _ _ _ _ _ _ _ _ _ _] -> w43
          tunnel: w41 -> [w48 w61 _ _ w103 w119 w134 w146 w163 w175 w187 w199 w211 w224 w237 w249 w262 w274 w289]
          tunnel: [w52 w65 w77 _ w104 w122 w135 w147 w153 w168 w180 w192 w204 w216 w229 w242 w254 w267 w282] -> w47
          tunnel: w42 -> [w49 w62 w75 w81 w102 w120 w132 w144 w161 w173 w185 w197 w209 w222 w235 w247 w260 w272 w287]
          event User Event {
            # "Another Module called the \"Show Panel\" API Method."
            n228 = event-data() -> ("Module ID"=w50:i32)  [unwired: 1 in]
            n229 = call "Addressed to This Module.vi"("Module ID from Argument"=w50, "Module Admin"=w49) -> ("Addressed to this instance?"=w51:bool)  [unwired: 8 in, 1 out]
            n230 = case shown="True" w51 {
              tunnel: w49 -> [_ w57]
              tunnel: w48 -> [_ w55]
              tunnel: [_ w60] -> w52
              frame False {
              }
              frame True {
                # "Show the panel of this VI, and send a status updated message to let listeners know."
                n231 = control-ref of="This VI"() -> (w59:refnum<vi>)
                n232 = property class="Mod Admin"(reference=w57) -> ("Accessors:Module ID"=w56:i32)  [unwired: 1 in, 2 out]
                n233 = call "Open VI Panel.vi"("VI"=w59) -> ()  [unwired: 10 in, 1 out]
                n234 = call-poly <vilib>:"Delacor_lib_QMH_Enqueue Message (poly).vi"("Message Data"=TRUE, "Message"="Panel Status" ("format string"), "Message Queue in"=w55) -> ("error out"=w60:errorcluster)  [unwired: 7 in, 1 out]
                n235 = call "Status Updated.vi"("Status"="Panel shown." ("format string"), "Module ID"=w56) -> ()  [unwired: 9 in, 1 out]
              }
            }
          }
          event User Event {
            # "Another Module called the \"Hide Panel\" API Method."
            n236 = event-data() -> ("Module ID"=w63:i32)  [unwired: 1 in]
            n237 = call "Addressed to This Module.vi"("Module ID from Argument"=w63, "Module Admin"=w62) -> ("Addressed to this instance?"=w64:bool)  [unwired: 8 in, 1 out]
            n238 = case shown="True" w64 {
              tunnel: w62 -> [_ w70]
              tunnel: w61 -> [_ w66]
              tunnel: [_ w73] -> w65
              frame False {
              }
              frame True {
                n239 = control-ref of="This VI"() -> (w72:refnum<vi>)
                n240 = property class="Mod Admin"(reference=w70) -> ("Accessors:Module ID"=w69:i32)  [unwired: 1 in, 2 out]
                n241 = call "Hide VI Panel.vi"("VI"=w72) -> ()  [unwired: 10 in, 1 out]
                n242 = call "Status Updated.vi"("Status"="Panel hidden." ("format string"), "Module ID"=w69) -> ()  [unwired: 9 in, 1 out]
                n243 = call-poly <vilib>:"Delacor_lib_QMH_Enqueue Message (poly).vi"("Message Data"=FALSE, "Message"="Panel Status" ("format string"), "Message Queue in"=w66) -> ("error out"=w73:errorcluster)  [unwired: 7 in, 1 out]
              }
            }
          }
          event User Event {
            # "For cloneable running as singleton, broadcast that the module is running."
            n244 = event-data() -> ("Module ID"=w74:i32)  [unwired: 1 in]
            n245 = call "Addressed to This Module.vi"("Module ID from Argument"=w74, "Module Admin"=w75) -> ("Addressed to this instance?"=w76:bool)  [unwired: 8 in, 1 out]
            n246 = case shown="True" w76 {
              tunnel: [_ w80] -> w77
              tunnel: w74 -> [_ w79]
              frame False {
              }
              frame True {
                n247 = call "Update Module Execution Status.vi"("Running?"=TRUE, "Module ID"=w79) -> ("error out"=w80:errorcluster)  [unwired: 9 in]
              }
            }
          }
          event User Event {
            # "Another Module called the \"Show Diagram\" API Method. This event is used for debugging."
            n248 = event-data() -> ("Module ID"=w82:i32)  [unwired: 1 in]
            n249 = call "Addressed to This Module.vi"("Module ID from Argument"=w82, "Module Admin"=w81) -> ("Addressed to this instance?"=w83:bool)  [unwired: 8 in, 1 out]
            n250 = case shown="True" w83 {
              tunnel: w81 -> [_ w84]
              frame False {
              }
              frame True {
                n251 = disable-structure shown="RUN_TIME_ENGINE==False" {
                  disable-tunnel: w84 -> [w85 _]
                  frame condition #0 (active) {
                    # "functionality not available in exe"
                    n252 = invoke class="VI" method="Lock State.Get"() -> (error out=w91:errorcluster, "Get Lock State"=w90:T4, "pwd in cache"=w87:bool)  [unwired: 4 in, 1 out]
                    n253 = Equal?(x=T4."Password-protected", y=w90) -> (x = y?=w88:bool)
                    n254 = Compound Arithmetic op=AND(w88, invert w87) -> (w86:bool)
                    n255 = case shown="False" w86 {
                      tunnel: w91 -> [w96 _]
                      tunnel: w85 -> [w93 _]
                      frame False {
                        n256 = property class="Mod Admin"(reference=w93) -> ("Accessors:Module ID"=w92:i32)  [unwired: 1 in, 2 out]
                        n257 = property class="VI"(error in=w96, "BDWin.Open"=TRUE ("Block Diagram Window:Open")) -> ()  [unwired: 1 in, 2 out]
                        n258 = call "Status Updated.vi"("Status"="Block Diagram shown." ("format string"), "Module ID"=w92) -> ()  [unwired: 9 in, 1 out]
                      }
                      frame True {
                        # "Password-protected VI, and the password is not in the cache. Do not show the diagram."
                      }
                    }
                  }
                  frame condition #1 {
                  }
                }
              }
            }
          }
          event User Event {
            # "Another Module called the \"Stop Module\" API Method  or the Message Handling Loop below."
            n259 = event-data() -> ("Module ID"=w98:i32, "Wait for Module to stop?"=w99:bool, "Origin"=w97:string)  [unwired: 1 in]
            n260 = call "Addressed to This Module.vi"("Module ID from Argument"=w98, "Module Admin"=w102) -> ("Addressed to this instance?"=w101:bool)  [unwired: 8 in, 1 out]
            n261 = case shown="True" w101 {
              tunnel: [_ w116] -> w104
              tunnel: w103 -> [_ w112]
              tunnel: [_ TRUE] -> w100
              tunnel: w99 -> [_ w107]
              tunnel: w98 -> [_ w109]
              tunnel: w97 -> [_ w105]
              frame False {
              }
              frame True {
                # "The event can get fired from the Exit message. The queue gets destroyed there. In this case, the Enqueue VI will return error 1. It is safe to ignore, because the module is already exiting."
                n262 = local write "Status"(w105) -> ()
                n263 = Bundle By Name(cluster=T5 {"Module ID"=-1, "Origin"="", "Exit via Stop Module Req?"=FALSE, "Wait for Module to stop?"=FALSE} ("Stop Argument"), "Module ID"=w109, "Exit via Stop Module Req?"=TRUE, "Wait for Module to stop?"=w107) -> (w106:T5)
                n264 = call-poly <vilib>:"Delacor_lib_QMH_Enqueue Message (poly).vi"("Priority Message? (F)"=TRUE, "Message Data"=w106, "Message"="Exit", "Message Queue in"=w112) -> ("error out"=w117:errorcluster)  [unwired: 6 in, 1 out]
                n265 = call <vilib>:"Clear Errors.vi"("error in (no error)"=w117, "specific error code to clear (0: all)"=1) -> ("error out"=w116:errorcluster)  [unwired: 4 in, 1 out]
              }
            }
          }
          event Panel Close? {
            w121 = TRUE  # Discard the event, the MHL is responsible for closing and stopping this VI.
            # "Hide the panel or send the 'Exit' message if the user clicks the 'X' on the module main VI panel."
            n266 = event-data() -> ()  [unwired: 1 in, 1 out]
            n267 = property class="Mod Admin"(reference=w120) -> ("Accessors:External Launch"=w118:bool)  [unwired: 1 in, 2 out]
            n268 = case shown="True" w118 {
              tunnel: w119 -> [_ w126]
              tunnel: [_ w127] -> w122
              frame True {
                # "If externally launched, clicking the 'X' hides the panel, but doesn't close it."
                n269 = control-ref of="This VI"() -> (w123:refnum<vi>)
                n270 = call "Hide VI Panel.vi"("VI"=w123) -> ()  [unwired: 10 in, 1 out]
              }
              frame False {
                # "If run as a stand-alone VI, clicking the panel 'X' stops the VI."
                n271 = call-poly <vilib>:"Delacor_lib_QMH_Enqueue Message (poly).vi"("Priority Message? (F)"=TRUE, "Message"="Exit", "Message Queue in"=w126) -> ("error out"=w127:errorcluster)  [unwired: 7 in, 1 out]
              }
            }
            n272 = event-data("Discard?"=w121) -> ()  [unwired: 1 in, 1 out]
          }
          event User Event {
            # "Another Module called the \"Draw Panel into Subpanel\" API Method."
            n273 = event-data() -> ("Module ID"=w129:i32, "Sub Panel"=w128:refnum<vi>)  [unwired: 1 in]
            n274 = Bundle(cluster=T6 {"Module ID"=-1, "Sub Panel"=refnum} ("Draw Panel into Subpanel Argument"), "Module ID"=w129, "Sub Panel"=w128) -> (w130:T6)
            n275 = call "Addressed to This Module.vi"("Module ID from Argument"=w129, "Module Admin"=w132) -> ("Addressed to this instance?"=w133:bool)  [unwired: 8 in, 1 out]
            n276 = case shown="True" w133 {
              tunnel: w134 -> [_ w138]
              tunnel: w130 -> [_ w136]
              tunnel: [_ w139] -> w135
              frame False {
              }
              frame True {
                n277 = call-poly <vilib>:"Delacor_lib_QMH_Enqueue Message (poly).vi"("Message Data"=w136, "Message"="Draw Panel into Subpanel", "Message Queue in"=w138) -> ("error out"=w139:errorcluster)  [unwired: 7 in, 1 out]
              }
            }
          }
          event User Event {
            # "Another Module called the \"Remove Panel from Subpanel\" API Method."
            n278 = event-data() -> ("Module ID"=w141:i32, "Boolean"=w140:bool)  [unwired: 1 in]
            n279 = Bundle(cluster=T7 {"Module ID"=-1, "Boolean"=FALSE} ("Remove Panel from Subpanel Argument"), "Module ID"=w141, "Boolean"=w140) -> (w142:T7)
            n280 = call "Addressed to This Module.vi"("Module ID from Argument"=w141, "Module Admin"=w144) -> ("Addressed to this instance?"=w145:bool)  [unwired: 8 in, 1 out]
            n281 = case shown="True" w145 {
              tunnel: w146 -> [_ w150]
              tunnel: w142 -> [_ w148]
              tunnel: [_ w151] -> w147
              frame False {
              }
              frame True {
                n282 = call-poly <vilib>:"Delacor_lib_QMH_Enqueue Message (poly).vi"("Message Data"=w148, "Message"="Remove Panel from Subpanel", "Message Queue in"=w150) -> ("error out"=w151:errorcluster)  [unwired: 7 in, 1 out]
              }
            }
          }
          event User Event {
            # "Another Module called the \"Connect\" API Method."
            n283 = event-data() -> ("Module ID"=w158:i32, "VISA resource name"=w157:refnum<visa-resource-name>, "Port config"=w156:T28, "Wait Notifier"=w155:refnum<notifier>, "wait for reply"=w154:bool, "Simulate?"=w152:bool)  [unwired: 1 in]
            n284 = Bundle(cluster=T8 {"Module ID"=-1, "VISA resource name"="", "Port config"={"baud rate"=9600, "data bits"=8, "parity"=enum."None", "stop bits"=10}, "Wait Notifier"=refnum, "wait for reply"=FALSE, "Simulate?"=FALSE} ("Connect Argument"), "Module ID"=w158, "VISA resource name"=w157, "Port config"=w156, "Wait Notifier"=w155, "wait for reply"=w154, "Simulate?"=w152) -> (w159:T8)
            n285 = call "Addressed to This Module.vi"("Module ID from Argument"=w158, "Module Admin"=w161) -> ("Addressed to this instance?"=w162:bool)  [unwired: 8 in, 1 out]
            n286 = case shown="True" w162 {
              tunnel: w163 -> [_ w167]
              tunnel: w159 -> [_ w165]
              tunnel: [_ w164] -> w153
              frame False {
              }
              frame True {
                n287 = call-poly <vilib>:"Delacor_lib_QMH_Enqueue Message (poly).vi"("Message Data"=w165, "Message"="Connect", "Message Queue in"=w167) -> ("error out"=w164:errorcluster)  [unwired: 7 in, 1 out]
              }
            }
          }
          event User Event {
            # "Another Module called the \"Move\" API Method."
            n288 = event-data() -> ("Module ID"=w170:i32, "Wavelength"=w169:dbl)  [unwired: 1 in]
            n289 = Bundle(cluster=T9 {"Module ID"=-1, "Wavelength"=0.0} ("Move Argument"), "Module ID"=w170, "Wavelength"=w169) -> (w171:T9)
            n290 = call "Addressed to This Module.vi"("Module ID from Argument"=w170, "Module Admin"=w173) -> ("Addressed to this instance?"=w174:bool)  [unwired: 8 in, 1 out]
            n291 = case shown="True" w174 {
              tunnel: w175 -> [_ w179]
              tunnel: w171 -> [_ w177]
              tunnel: [_ w176] -> w168
              frame False {
              }
              frame True {
                n292 = call-poly <vilib>:"Delacor_lib_QMH_Enqueue Message (poly).vi"("Message Data"=w177, "Message"="Move", "Message Queue in"=w179) -> ("error out"=w176:errorcluster)  [unwired: 7 in, 1 out]
              }
            }
          }
          event User Event {
            # "Another Module called the \"Read continuously\" API Method."
            n293 = event-data() -> ("Module ID"=w182:i32, "Timeout"=w181:i32)  [unwired: 1 in]
            n294 = Bundle(cluster=T10 {"Module ID"=-1, "Timeout"=0} ("Read continuously Argument"), "Module ID"=w182, "Timeout"=w181) -> (w183:T10)
            n295 = call "Addressed to This Module.vi"("Module ID from Argument"=w182, "Module Admin"=w185) -> ("Addressed to this instance?"=w186:bool)  [unwired: 8 in, 1 out]
            n296 = case shown="True" w186 {
              tunnel: w187 -> [_ w191]
              tunnel: w183 -> [_ w189]
              tunnel: [_ w188] -> w180
              frame False {
              }
              frame True {
                n297 = call-poly <vilib>:"Delacor_lib_QMH_Enqueue Message (poly).vi"("Message Data"=w189, "Message"="Read continuously", "Message Queue in"=w191) -> ("error out"=w188:errorcluster)  [unwired: 7 in, 1 out]
              }
            }
          }
          event User Event {
            # "Another Module called the \"Stop continous reading\" API Method."
            n298 = event-data() -> ("Module ID"=w194:i32, "Boolean"=w193:bool)  [unwired: 1 in]
            n299 = Bundle(cluster=T11 {"Module ID"=-1, "Boolean"=FALSE} ("Stop continous reading Argument"), "Module ID"=w194, "Boolean"=w193) -> (w195:T11)
            n300 = call "Addressed to This Module.vi"("Module ID from Argument"=w194, "Module Admin"=w197) -> ("Addressed to this instance?"=w198:bool)  [unwired: 8 in, 1 out]
            n301 = case shown="True" w198 {
              tunnel: w199 -> [_ w203]
              tunnel: w195 -> [_ w201]
              tunnel: [_ w200] -> w192
              frame False {
              }
              frame True {
                n302 = call-poly <vilib>:"Delacor_lib_QMH_Enqueue Message (poly).vi"("Message Data"=w201, "Message"="Stop continous reading", "Message Queue in"=w203) -> ("error out"=w200:errorcluster)  [unwired: 7 in, 1 out]
              }
            }
          }
          event User Event {
            # "Another Module called the \"Stop movement\" API Method."
            n303 = event-data() -> ("Module ID"=w206:i32, "Boolean"=w205:bool)  [unwired: 1 in]
            n304 = Bundle(cluster=T12 {"Module ID"=-1, "Boolean"=FALSE} ("Stop movement Argument"), "Module ID"=w206, "Boolean"=w205) -> (w207:T12)
            n305 = call "Addressed to This Module.vi"("Module ID from Argument"=w206, "Module Admin"=w209) -> ("Addressed to this instance?"=w210:bool)  [unwired: 8 in, 1 out]
            n306 = case shown="True" w210 {
              tunnel: w211 -> [_ w215]
              tunnel: w207 -> [_ w213]
              tunnel: [_ w212] -> w204
              frame False {
              }
              frame True {
                n307 = call-poly <vilib>:"Delacor_lib_QMH_Enqueue Message (poly).vi"("Message Data"=w213, "Message"="Stop movement", "Message Queue in"=w215) -> ("error out"=w212:errorcluster)  [unwired: 7 in, 1 out]
              }
            }
          }
          event User Event {
            # "Another Module called the \"Ask position\" API Method."
            n308 = event-data() -> ("Module ID"=w219:i32, "Wait Notifier"=w218:refnum<notifier>, "wait for reply"=w217:bool)  [unwired: 1 in]
            n309 = Bundle(cluster=T13 {"Module ID"=-1, "Wait Notifier"=refnum, "wait for reply"=FALSE} ("Ask position Argument"), "Module ID"=w219, "Wait Notifier"=w218, "wait for reply"=w217) -> (w220:T13)
            n310 = call "Addressed to This Module.vi"("Module ID from Argument"=w219, "Module Admin"=w222) -> ("Addressed to this instance?"=w223:bool)  [unwired: 8 in, 1 out]
            n311 = case shown="True" w223 {
              tunnel: w224 -> [_ w228]
              tunnel: w220 -> [_ w226]
              tunnel: [_ w225] -> w216
              frame False {
              }
              frame True {
                n312 = call-poly <vilib>:"Delacor_lib_QMH_Enqueue Message (poly).vi"("Message Data"=w226, "Message"="Ask position", "Message Queue in"=w228) -> ("error out"=w225:errorcluster)  [unwired: 7 in, 1 out]
              }
            }
          }
          event User Event {
            # "Another Module called the \"Position reached\" API Method."
            n313 = event-data() -> ("Module ID"=w232:i32, "Wait Notifier"=w231:refnum<notifier>, "wait for reply"=w230:bool)  [unwired: 1 in]
            n314 = Bundle(cluster=T14 {"Module ID"=-1, "Wait Notifier"=refnum, "wait for reply"=FALSE} ("Position reached Argument"), "Module ID"=w232, "Wait Notifier"=w231, "wait for reply"=w230) -> (w233:T14)
            n315 = call "Addressed to This Module.vi"("Module ID from Argument"=w232, "Module Admin"=w235) -> ("Addressed to this instance?"=w236:bool)  [unwired: 8 in, 1 out]
            n316 = case shown="True" w236 {
              tunnel: w237 -> [_ w241]
              tunnel: w233 -> [_ w239]
              tunnel: [_ w238] -> w229
              frame False {
              }
              frame True {
                n317 = call-poly <vilib>:"Delacor_lib_QMH_Enqueue Message (poly).vi"("Message Data"=w239, "Message"="Position reached", "Message Queue in"=w241) -> ("error out"=w238:errorcluster)  [unwired: 7 in, 1 out]
              }
            }
          }
          event User Event {
            # "Another Module called the \"Set speed\" API Method."
            n318 = event-data() -> ("Module ID"=w244:i32, "nm/min"=w243:dbl)  [unwired: 1 in]
            n319 = Bundle(cluster=T15 {"Module ID"=-1, "nm/min"=0.0} ("Set speed Argument"), "Module ID"=w244, "nm/min"=w243) -> (w245:T15)
            n320 = call "Addressed to This Module.vi"("Module ID from Argument"=w244, "Module Admin"=w247) -> ("Addressed to this instance?"=w248:bool)  [unwired: 8 in, 1 out]
            n321 = case shown="True" w248 {
              tunnel: w249 -> [_ w253]
              tunnel: w245 -> [_ w251]
              tunnel: [_ w250] -> w242
              frame False {
              }
              frame True {
                n322 = call-poly <vilib>:"Delacor_lib_QMH_Enqueue Message (poly).vi"("Message Data"=w251, "Message"="Set speed", "Message Queue in"=w253) -> ("error out"=w250:errorcluster)  [unwired: 7 in, 1 out]
              }
            }
          }
          event User Event {
            # "Another Module called the \"Get speed\" API Method."
            n323 = event-data() -> ("Module ID"=w257:i32, "Wait Notifier"=w256:refnum<notifier>, "wait for reply"=w255:bool)  [unwired: 1 in]
            n324 = Bundle(cluster=T16 {"Module ID"=-1, "Wait Notifier"=refnum, "wait for reply"=FALSE} ("Get speed Argument"), "Module ID"=w257, "Wait Notifier"=w256, "wait for reply"=w255) -> (w258:T16)
            n325 = call "Addressed to This Module.vi"("Module ID from Argument"=w257, "Module Admin"=w260) -> ("Addressed to this instance?"=w261:bool)  [unwired: 8 in, 1 out]
            n326 = case shown="True" w261 {
              tunnel: w262 -> [_ w266]
              tunnel: w258 -> [_ w264]
              tunnel: [_ w263] -> w254
              frame False {
              }
              frame True {
                n327 = call-poly <vilib>:"Delacor_lib_QMH_Enqueue Message (poly).vi"("Message Data"=w264, "Message"="Get speed", "Message Queue in"=w266) -> ("error out"=w263:errorcluster)  [unwired: 7 in, 1 out]
              }
            }
          }
          event User Event {
            # "Another Module called the \"Disconnect\" API Method."
            n328 = event-data() -> ("Module ID"=w269:i32, "Boolean"=w268:bool)  [unwired: 1 in]
            n329 = Bundle(cluster=T17 {"Module ID"=-1, "Boolean"=FALSE} ("Disconnect Argument"), "Module ID"=w269, "Boolean"=w268) -> (w270:T17)
            n330 = call "Addressed to This Module.vi"("Module ID from Argument"=w269, "Module Admin"=w272) -> ("Addressed to this instance?"=w273:bool)  [unwired: 8 in, 1 out]
            n331 = case shown="True" w273 {
              tunnel: w274 -> [_ w278]
              tunnel: w270 -> [_ w276]
              tunnel: [_ w275] -> w267
              frame False {
              }
              frame True {
                n332 = call-poly <vilib>:"Delacor_lib_QMH_Enqueue Message (poly).vi"("Message Data"=w276, "Message"="Disconnect", "Message Queue in"=w278) -> ("error out"=w275:errorcluster)  [unwired: 7 in, 1 out]
              }
            }
          }
          event User Event {
            # "Another Module called the \"Move (GOTO)\" API Method."
            n333 = event-data() -> ("Module ID"=w284:i32, "Position"=w283:dbl, "Echo?"=w281:bool, "Wait Notifier"=w280:refnum<notifier>, "wait for reply"=w279:bool)  [unwired: 1 in]
            n334 = call "Addressed to This Module.vi"("Module ID from Argument"=w284, "Module Admin"=w287) -> ("Addressed to this instance?"=w288:bool)  [unwired: 8 in, 1 out]
            n335 = Bundle(cluster=T18 {"Module ID"=-1, "Position"=0.0, "Echo?"=FALSE, "Wait Notifier"=refnum, "wait for reply"=FALSE} ("Move (GOTO) Argument"), "Module ID"=w284, "Position"=w283, "Echo?"=w281, "Wait Notifier"=w280, "wait for reply"=w279) -> (w285:T18)
            n336 = case shown="True" w288 {
              tunnel: w289 -> [_ w293]
              tunnel: w285 -> [_ w291]
              tunnel: [_ w290] -> w282
              frame False {
              }
              frame True {
                n337 = call-poly <vilib>:"Delacor_lib_QMH_Enqueue Message (poly).vi"("Message Data"=w291, "Message"="Move (GOTO)", "Message Queue in"=w293) -> ("error out"=w290:errorcluster)  [unwired: 7 in, 1 out]
              }
            }
          }
        }
        n338 = call-dynamic "Delacor_lib_QMH_Error Handler - Event Handling Loop.vi"("error in"=w47, "Message Queue in"=w41) -> ("dup error in"=w46:errorcluster)  [unwired: 8 in, 1 out]
      }
    }
    frame Error {
      n339 = call "Synchronize Caller Events.vi"("Module Admin"=w901) -> ("Module Admin out"=w900:refnum<class "Delacor_lib_QMH_Cloneable Module Admin.lvclass">)  [unwired: 9 in, 1 out]
      n340 = property class="Mod Admin"(reference=w900) -> ("Accessors:Module ID"=w899:i32)  [unwired: 1 in, 2 out]
      n341 = call-dynamic "Delacor_lib_QMH_Release Message Queue.vi"("error in"=w907, "Message Queue"=w898) -> ("error out"=w906:errorcluster)  [unwired: 9 in]
      n342 = call "Module Name--constant.vi"("Module ID"=w899) -> ("Module Name"=w904:string)  [unwired: 10 in]
      n343 = Format Into String(format string="An error occurred during initialization. %s is no longer running.", w904) -> (resulting string=w902:string)  [unwired: 2 in, 1 out]
      n344 = call "Error Reported.vi"("Additional Information"=w902, "Error"=w906, "Module ID"=w899) -> ()  [unwired: 8 in, 1 out]
    }
  }
  n345 = Merge Errors(w25, w24, w17) -> (w26:errorcluster)
  n346 = Unregister For Events(event registration refnum=w6) -> (error out=w15:errorcluster)  [unwired: 1 in]
  n347 = call "Close Module.vi"("error in"=w26, "Wait for stop?"=w8, "Module Admin in"=w10) -> ("error out"=w22:errorcluster, "External Launch"=w7:bool, "Module Admin out"=w9:refnum<class "Delacor_lib_QMH_Cloneable Module Admin.lvclass">)  [unwired: 6 in]
  n348 = call "Destroy Local Events.vi"("error in"=w15, "Local Events"=w1) -> ()  [unwired: 9 in, 1 out]
  n349 = Unregister For Events(event registration refnum=w14, error in=w22) -> (error out=w21:errorcluster)
  "error out" <- w21
  n350 = local write "Module Admin"(w9) -> ()
  n351 = case "External Launch?" shown="True" w7 {
    tunnel: w21 -> [_ w908]
    frame False {
    }
    frame True {
      n352 = case shown="No Error" w908 {
        frame No Error {
          n353 = invoke class="VI" method="FP.Close"() -> ()  [unwired: 3 in, 3 out]
        }
        frame Error {
          n354 = invoke class="VI" method="FP.Open"("Activate"=TRUE ("Activate?")) -> ()  [unwired: 4 in, 5 out]
        }
      }
    }
  }
